vi "LVSreadparams.vi"(0 "Port In":refnum<visa-resource-name>="ASRL18::INSTR", 3 "var query":string="frETWIUdmxlust[]^knXcwFqAPORj*<>,/b;:UdmD~T", 7 "error in":errorcluster, 11 "Get F&A":bool, 12 "Prog Chan?":bool, 14 "ChSt":bool) -> (1 "RFonA":bool, 2 "RFonB":bool, 4 "LevA":bool, 5 "LevB":bool, 8 "FchA":dbl, 9 "FchB":dbl, 13 "ComError":bool, 16 "AdBm":dbl, 17 "BdBm":dbl, 20 "Port Out":refnum<visa-resource-name>="ASRL18::INSTR", 21 "NowLevel":bool, 23 "cluster":T1, 24 "NowFreq":dbl, 25 "NowdBm":dbl, 27 "error out":errorcluster)   [LabVIEW 2013]
uses:
  <vilib>/Utility/error.llb/DialogType.ctl
  instr.lib/lvserial/lvserial.lvlib
panel:
  out "NowRFon":bool
  out "result":i32
  out "element":dbl
  out "Array":dbl[](array[numeric])
  out "output":string="C1f?a?C0"
  # "Ch 0(A)"
  # "Ch1(B)"
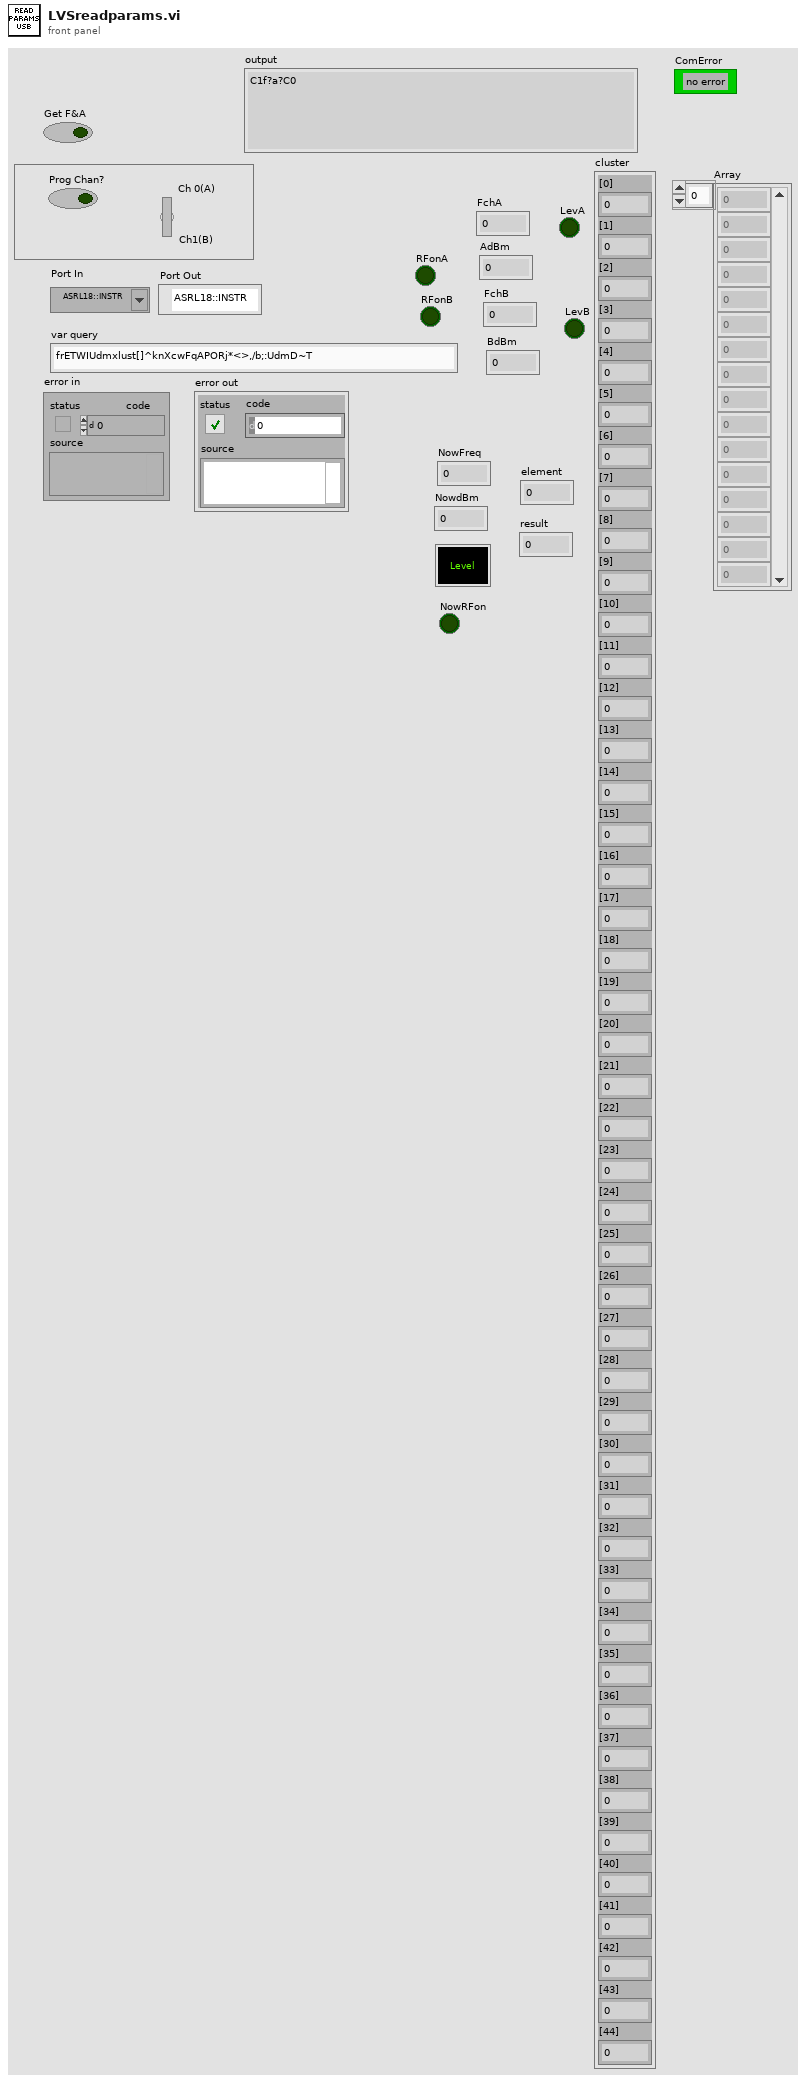
[diagram p1: front panel]
types:
  T1 = cluster{"[0]":dbl, "[1]":dbl, "[2]":dbl, "[3]":dbl, "[4]":dbl, "[5]":dbl, "[6]":dbl, "[7]":dbl, "[8]":dbl, "[9]":dbl, "[10]":dbl, "[11]":dbl, "[12]":dbl, "[13]":dbl, "[14]":dbl, "[15]":dbl, "[16]":dbl, "[17]":dbl, "[18]":dbl, "[19]":dbl, "[20]":dbl, "[21]":dbl, "[22]":dbl, "[23]":dbl, "[24]":dbl, "[25]":dbl, "[26]":dbl, "[27]":dbl, "[28]":dbl, "[29]":dbl, "[30]":dbl, "[31]":dbl, "[32]":dbl, "[33]":dbl, "[34]":dbl, "[35]":dbl, "[36]":dbl, "[37]":dbl, "[38]":dbl, "[39]":dbl, "[40]":dbl, "[41]":dbl, "[42]":dbl, "[43]":dbl, "[44]":dbl}
  T2 = typedef "DialogType.ctl" = u16
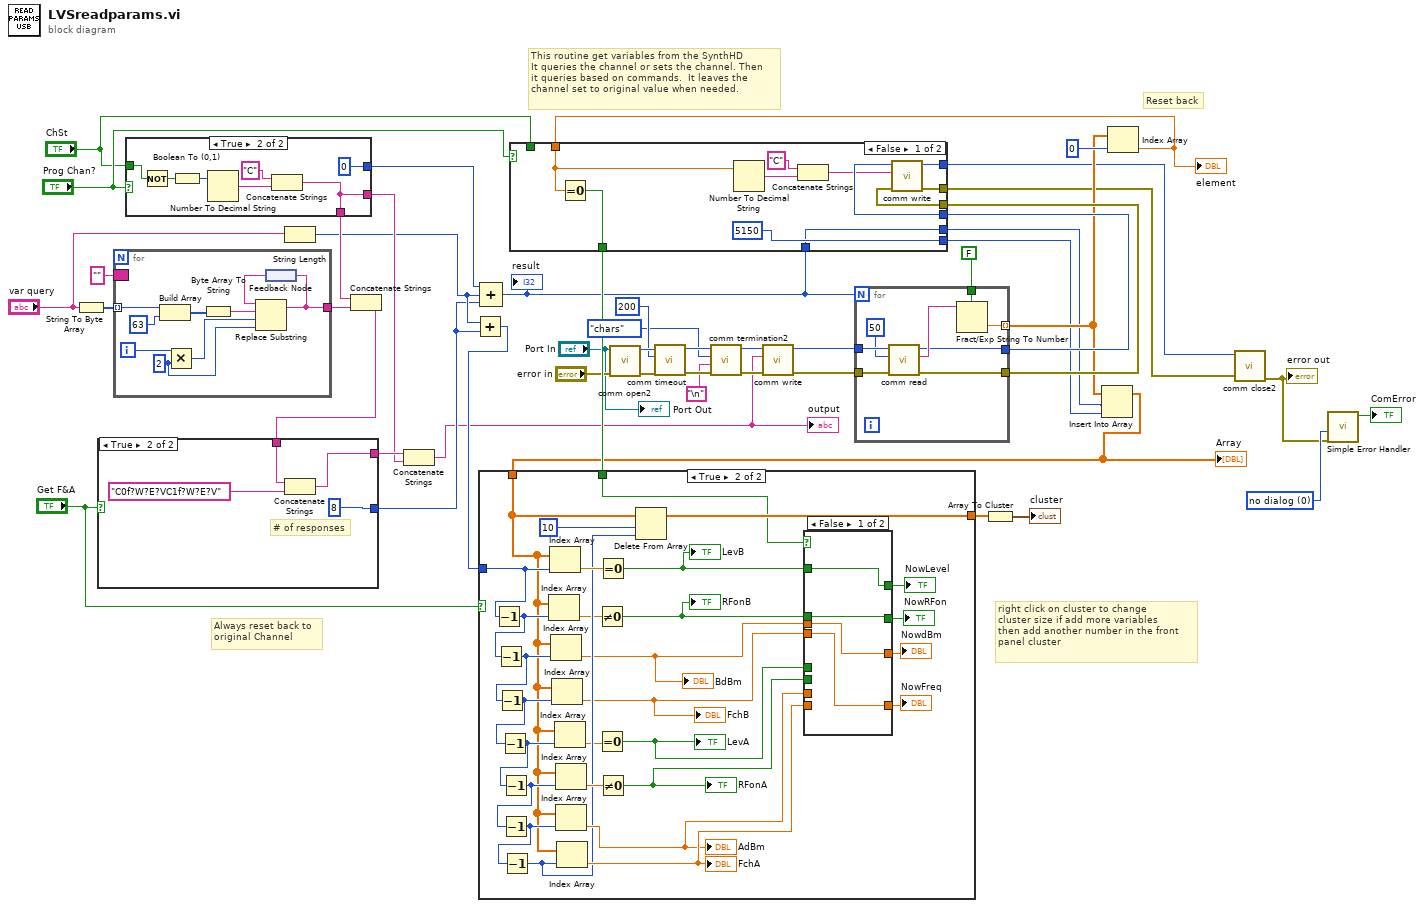
[diagram p0: block diagram]
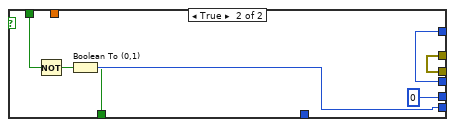
[diagram p2: hidden frame]
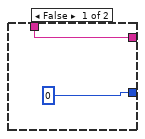
[diagram p5: hidden frame]
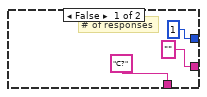
[diagram p6: hidden frame]
diagram:
  w19 = T2 0 items=["no dialog", "OK message", "continue or stop message", "OK message + warnings", "continue/stop + warnings"] ("type of dialog (OK msg:1)")
  # "right click on cluster to change\ncluster size if add more variables\nthen add another number in the front\npanel cluster"
  # "This routine get variables from the SynthHD\nIt queries the channel or sets the channel. Then\nit queries based on commands.  It leaves the\nchannel set to original value when needed."
  # "Reset back"
  # "Always reset back to\noriginal Channel"
  n1 = String To Byte Array(string="var query") -> (unsigned byte array=w46:u8[])
  n2 = for {
    tunnel: w46 -> [w56] mode=indexing
    tunnel: [w48] -> w44
    border: "" ("result string") -> [_]
    i -> [w52]
    w50 = 2 ("y")
    n3 = Build Array(w56, u8 63 ("element")) -> (w54:u8[])
    n4 = Multiply(x=w52, y=w50) -> (x*y=w51:i32)
    n5 = Byte Array To String(unsigned byte array=w54) -> (string=w53:string)
    n6 = feedback #1() -> (w49:string)
    n7 = Replace Substring(2:w50, 3:w51, 4:w53, 5:w49) -> (1:w48:string)  [unwired: 1 out]
    n8 = feedback-in #1(w48) -> ()
  }
  n9 = case shown="True" "Prog Chan?" {
    tunnel: ["C?" ("string") w61] -> w43
    tunnel: "ChSt" -> [_ w63]
    tunnel: ["" w61] -> w39
    tunnel: [1 ("y") 0 ("y")] -> w29
    frame False {
      # "# of responses"
    }
    frame True {
      n10 = Not(x=w63) -> (.not. x?=w62:bool)
      n11 = Boolean To (0,1)(Boolean=w62) -> (0, 1=w66:i16)
      n12 = Number To Decimal String(number=w66) -> (decimal integer string=w65:string)  [unwired: 1 in]
      n13 = Concatenate Strings("C" ("element"), w65) -> (w61:string)
    }
  }
  n14 = String Length(string="var query") -> (length=w23:i32)
  n15 = Concatenate Strings(w43, w44) -> (w42:string)
  n16 = case shown="True" "Get F&A" {
    tunnel: [w67 w69] -> w40
    tunnel: [0 ("y") 8 ("y")] -> w21
    tunnel: w42 -> [w67 w70]
    frame False {
    }
    frame True {
      # "# of responses"
      n17 = Concatenate Strings(w70, "C0f?W?E?VC1f?W?E?V" ("string")) -> (w69:string)
    }
  }
  n18 = Concatenate Strings(w40, w39) -> (w8:string)
  "output" <- w8
  n19 = Add(x=w23, y=w21) -> (x+y=w22:i32)
  n20 = Compound Arithmetic op=ADD(w29, w23, w21) -> (w24:i32)
  "result" <- w24
  n21 = call "comm open2.vi"("error in (no error)"="error in", "Comm Port Name"="Port In") -> ("error out"=w17:errorcluster, "Comm Handle"=w16:u32)  [unwired: 3 in, 1 out]
  n22 = call "comm timeout.vi"("error in (no error)"=w17, "Timeout"=u32 200 ("timeout (10sec)"), "Comm Handle"=w16) -> ("error out"=w14:errorcluster, "dup Comm Handle"=w13:u32)  [unwired: 7 in]
  n23 = call "comm termination2.vi"("error in (no error)"=w14, "termination"="\n", "Termination Mode"=enum16{"none", "chars", "string", "regex"}."chars", "Comm Handle"=w13) -> ("error out"=w9:errorcluster, "dup Comm Handle"=w10:u32)  [unwired: 6 in]
  n24 = call "comm write.vi"("error in (no error)"=w9, "string to write"=w8, "Comm Handle"=w10) -> ("error out"=w6:errorcluster, "dup Comm Handle"=w7:u32)  [unwired: 6 in, 1 out]
  n25 = for {
    N: w24 -> [_]
    tunnel: w6 -> [w77]
    tunnel: w7 -> [w78]
    tunnel: [w73] -> w32
    tunnel: [w74] -> w33
    tunnel: [w80] -> w28 mode=indexing
    tunnel: FALSE ("use system decimal point (T)") -> [w79]
    n26 = call "comm read.vi"("error in (no error)"=w77, "requested byte count"=u32 50 ("byte count"), "Comm Handle"=w78) -> ("error out"=w74:errorcluster, "string read"=w75:string, "dup Comm Handle"=w73:u32)  [unwired: 5 in, 1 out]
    n27 = Fract/Exp String To Number(use system decimal point (T)=w79, string=w75) -> (number=w80:dbl)  [unwired: 2 in, 1 out]
  }
  n28 = Index Array(array=w28, index=0) -> (element=w30:dbl)
  "element" <- w30
  n29 = case shown="False" "Prog Chan?" {
    tunnel: "ChSt" -> [_ w92]
    tunnel: [w91 w92] -> w35
    tunnel: w30 -> [w88 _]
    tunnel: w32 -> [w83 w96]
    tunnel: w33 -> [w84 w97]
    tunnel: [w85 w97] -> w5
    tunnel: [w81 w96] -> w3
    tunnel: [w86 0 ("y")] -> w26
    tunnel: [5150 ("y") w94] -> w25
    tunnel: w24 -> [w86 _]
    frame False {
      n30 = Equal To 0?(x=w88) -> (x = 0?=w91:bool)
      n31 = Number To Decimal String(number=w88) -> (decimal integer string=w90:string)  [unwired: 1 in]
      n32 = Concatenate Strings("C" ("element"), w90) -> (w82:string)
      n33 = call "comm write.vi"("error in (no error)"=w84, "string to write"=w82, "Comm Handle"=w83) -> ("error out"=w85:errorcluster, "dup Comm Handle"=w81:u32)  [unwired: 6 in, 1 out]
    }
    frame True {
      n34 = Not(x=w92) -> (.not. x?=w93:bool)
      n35 = Boolean To (0,1)(Boolean=w93) -> (0, 1=w94:i16)
    }
  }
  n36 = Insert Into Array(array=w28, index=w26, new element=w25) -> (w27:dbl[])
  "Array" <- w27
  n37 = case shown="True" "Get F&A" {
    tunnel: w27 -> [w98 w112]
    tunnel: w22 -> [_ w122]
    tunnel: [w98 w124] -> w34
    tunnel: w35 -> [_ w118]
    frame False {
    }
    frame True {
      n38 = Decrement(x=w122) -> (x-1=w126:i32)
      n39 = Decrement(x=w126) -> (x-1=w125:i32)
      n40 = Decrement(x=w125) -> (x-1=w117:i32)
      n41 = Decrement(x=w117) -> (x-1=w116:i32)
      n42 = Decrement(x=w116) -> (x-1=w114:i32)
      n43 = Decrement(x=w114) -> (x-1=w113:i32)
      n44 = Decrement(x=w113) -> (x-1=w108:i32)
      n45 = Index Array(array=w112, index=w126) -> (element=w101:dbl)
      n46 = Index Array(array=w112, index=w122) -> (element=w115:dbl)
      n47 = Index Array(array=w112, index=w125) -> (element=w102:dbl)
      "BdBm" <- w102
      n48 = Index Array(array=w112, index=w117) -> (element=w103:dbl)
      "FchB" <- w103
      n49 = Index Array(array=w112, index=w116) -> (element=w107:dbl)
      n50 = Index Array(array=w112, index=w114) -> (element=w109:dbl)
      n51 = Index Array(array=w112, index=w113) -> (element=w110:dbl)
      "AdBm" <- w110
      n52 = Index Array(array=w112, index=w108) -> (element=w111:dbl)
      "FchA" <- w111
      n53 = Not Equal To 0?(x=w101) -> (x != 0?=w100:bool)
      "RFonB" <- w100
      n54 = Equal To 0?(x=w107) -> (x = 0?=w104:bool)
      "LevA" <- w104
      n55 = Equal To 0?(x=w115) -> (x = 0?=w99:bool)
      "LevB" <- w99
      n56 = Not Equal To 0?(x=w109) -> (x != 0?=w105:bool)
      "RFonA" <- w105
      n57 = Delete From Array(array=w112, length=10, index=w108) -> (array with subset deleted=w124:dbl[])  [unwired: 1 out]
      n58 = case shown="False" w118 {
        tunnel: [w129 w134] -> w120
        tunnel: [w130 w133] -> w121
        tunnel: [w127 w131] -> w119
        tunnel: w110 -> [_ w134]
        tunnel: w111 -> [_ w133]
        tunnel: [w128 w132] -> w106
        tunnel: w105 -> [_ w132]
        tunnel: w104 -> [_ w131]
        tunnel: w103 -> [w130 _]
        tunnel: w102 -> [w129 _]
        tunnel: w100 -> [w128 _]
        tunnel: w99 -> [w127 _]
        frame False {
        }
        frame True {
        }
      }
      "NowdBm" <- w120
      "NowFreq" <- w121
      "NowLevel" <- w119
      "NowRFon" <- w106
    }
  }
  n59 = Array To Cluster(array=w34) -> (cluster=→"cluster":T1)
  n60 = call "comm close2.vi"("error in (no error)"=w5, "Comm Handle"=w3) -> ("error out"=w4:errorcluster)  [unwired: 5 in]
  "error out" <- w4
  n61 = call <vilib>:"Simple Error Handler.vi"("type of dialog (OK msg:1)"=w19, "error in (no error)"=w4) -> ("error?"=→"ComError":bool)  [unwired: 7 out]
  "Port Out" <- "Port In"
